vi "InjB-RT.vi"() -> ()   [LabVIEW 2016]
uses:
  <vilib>/rvi/interface/nirviOpenFPGA/nirviOpenFPGA.xnode
  InjB-FPGA.vi
  <vilib>/rvi/interface/nirviReadWriteControl/nirviReadWriteControl.xnode
  HV Readbacks.ctl
  RT ctls.lvlib
  <vilib>/Utility/error.llb/Error Cluster From Error Code.vi
  <vilib>/rvi/interface/Simulation/niFpgaSimulationCallBeginRW.vi
  <vilib>/rvi/errors/niLvFpgaAdjustHostInterfaceError.vi
  Aperture RT Readbacks.ctl
  <vilib>/platform/TimedLoop/XDataNode/XDataNode.xnode
  <vilib>/Platform/TimedLoop/XDataNode/nitl_modes.ctl
  <vilib>/Platform/TimedLoop/XDataNode/XDNodeRunTimeDep.lvlib
  <vilib>/Platform/TimedLoop/XDataNode/wakeup.ctl
  <vilib>/Platform/TimedLoop/XDataNode/timing_clust.ctl
  Glassman Control.ctl
  NiFpgaLv.dll
  Pressure Gauge.ctl
  HV Controls.ctl
  Aperture RT Controls.ctl
panel:
  out "Cryo ON-Time RAW":string
  out "Cryo 1st Stage Temperature RAW":string
  out "Cryo 1st Stage Temperature":string
  out "Cryo ON-Time":string
  out "Cryo Status":string
  out "Cryo Status RAW":string
  out "Beamline":T1
  out "Ion Source":T1
  out "Ion Source IG2":dbl
  out "Ion Source CG2":dbl
  out "Ion Source CG1":dbl
  out "Ion Source IG1":dbl
  out "Beamline IG1":dbl
  out "Beamline CG1":dbl
  out "Beamline IG2":dbl
  out "Beamline CG2":dbl
  in  "Injector Aperture Controls":T2
  in  "Injector HV Controls":T3
  out "Injector Aperture Readbacks":T4
  out "Injector HV Readbacks":T5
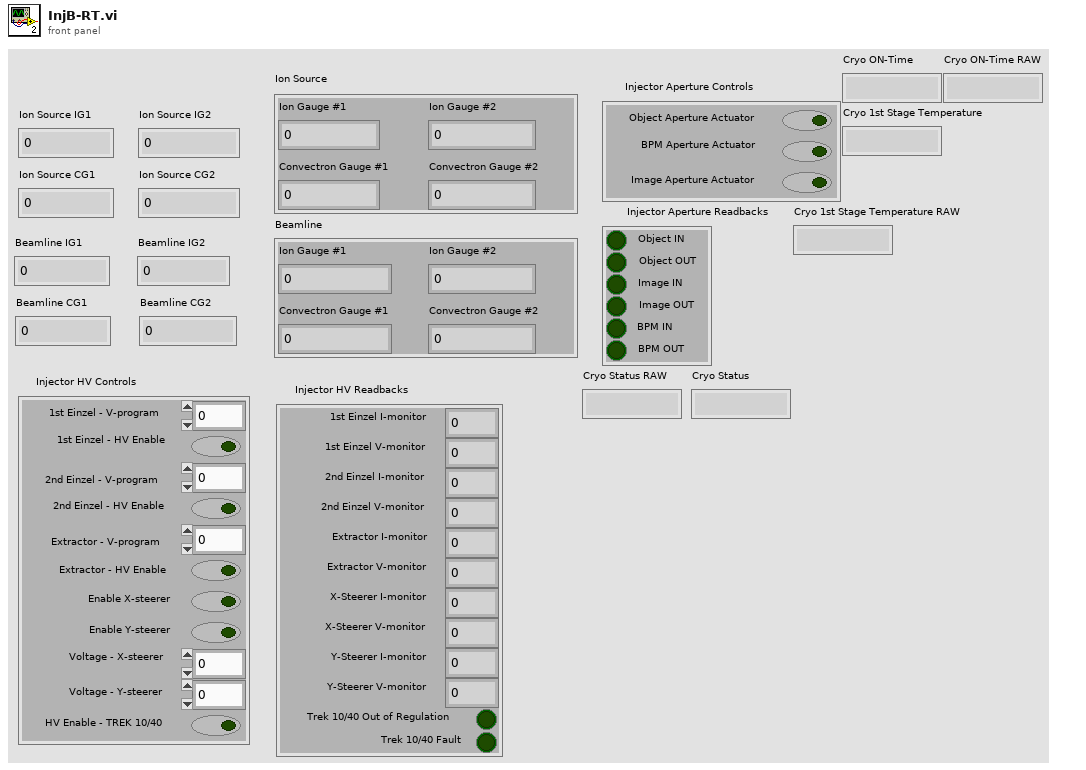
[diagram p1: front panel]
types:
  T1 = typedef "Pressure Gauge.ctl" = cluster{"Ion Gauge #1":dbl, "Convectron Gauge #1":dbl, "Convectron Gauge #2":dbl, "Ion Gauge #2":dbl}
  T2 = typedef "RT ctls.lvlib/Aperture RT Controls.ctl" = cluster{"Object Aperture Actuator":bool, "BPM Aperture Actuator":bool, "Image Aperture Actuator":bool}
  T3 = typedef "RT ctls.lvlib/HV Controls.ctl" = cluster{"Enable X-steerer":bool, "Enable Y-steerer":bool, "Voltage - X-steerer":fxp<+/-,20,5>, "Voltage - Y-steerer":fxp<+/-,20,5>, "HV Enable - TREK 10/40":bool, "1st Einzel - V-program":fxp<+/-,20,5>, "1st Einzel - HV Enable":bool, "2nd Einzel - V-program":fxp<+/-,20,5>, "2nd Einzel - HV Enable":bool, "Extractor - V-program":fxp<+/-,20,5>, "Extractor - HV Enable":bool}
  T4 = typedef "RT ctls.lvlib/Aperture RT Readbacks.ctl" = cluster{"Object IN":bool, "Object OUT":bool, "Image IN":bool, "Image OUT":bool, "BPM IN":bool, "BPM OUT":bool}
  T5 = typedef "RT ctls.lvlib/HV Readbacks.ctl" = cluster{"1st Einzel I-monitor":fxp<+/-,26,5>, "1st Einzel V-monitor":fxp<+/-,26,5>, "2nd Einzel I-monitor":fxp<+/-,26,5>, "2nd Einzel V-monitor":fxp<+/-,26,5>, "Extractor I-monitor":fxp<+/-,26,5>, "Extractor V-monitor":fxp<+/-,26,5>, "X-Steerer I-monitor":fxp<+/-,26,5>, "X-Steerer V-monitor":fxp<+/-,26,5>, "Y-Steerer I-monitor":fxp<+/-,26,5>, "Y-Steerer V-monitor":fxp<+/-,26,5>, "Trek 10/40 Out of Regulation":bool, "Trek 10/40 Fault":bool}
  T6 = typedef "XDNodeRunTimeDep.lvlib/timing_clust.ctl" = cluster{"Expected End [f-1]":u64, "Actual End [f-1]":u64, "Finished Late? [f-1]":bool, "Expected End [i-1]":u64, "Actual End [i-1]":u64, "Finished Late? [i-1]":bool, "Expected Start [i]":u64, "Actual Start [i]":u64, "Expected Start [f]":u64, "Actual Start [f]":u64, "Source Name":string, "Structure Name":string, "Period":i64, "Deadline":i64, "Offset":i64, "Start":i64, "Priority":i32, "Timeout":i32, "Mode":T7, "Wakeup Reason":T8, "Error":errorcluster, "Source Type":string, "Secondary Source Type":string, "Global End Time":u64, "Global Start Time":u64, "Frame Duration":u64, "Iteration Duration":u64, "Assigned CPU":i32, "I/O Scan Engine Mode":u32}
  T7 = typedef "XDNodeRunTimeDep.lvlib/nitl_modes.ctl" = enum32{"No Change", "Process missed periods, maintain original phase", "Discard missed periods, maintain original phase", "Process missed periods, ignore original phase", "Discard missed periods, ignore original phase"}
  T8 = typedef "XDNodeRunTimeDep.lvlib/wakeup.ctl" = enum32{"Normal", "Aborted", "Asynchronous wakeup", "Timing source error", "Timed loop error", "Timeout"}
  T9 = cluster{"I-monitor":fxp<+/-,26,5>, "V-monitor":fxp<+/-,26,5>}
  T10 = typedef "Glassman Control.ctl" = cluster{"V-program":fxp<+/-,20,5>, "HV Enable":bool}
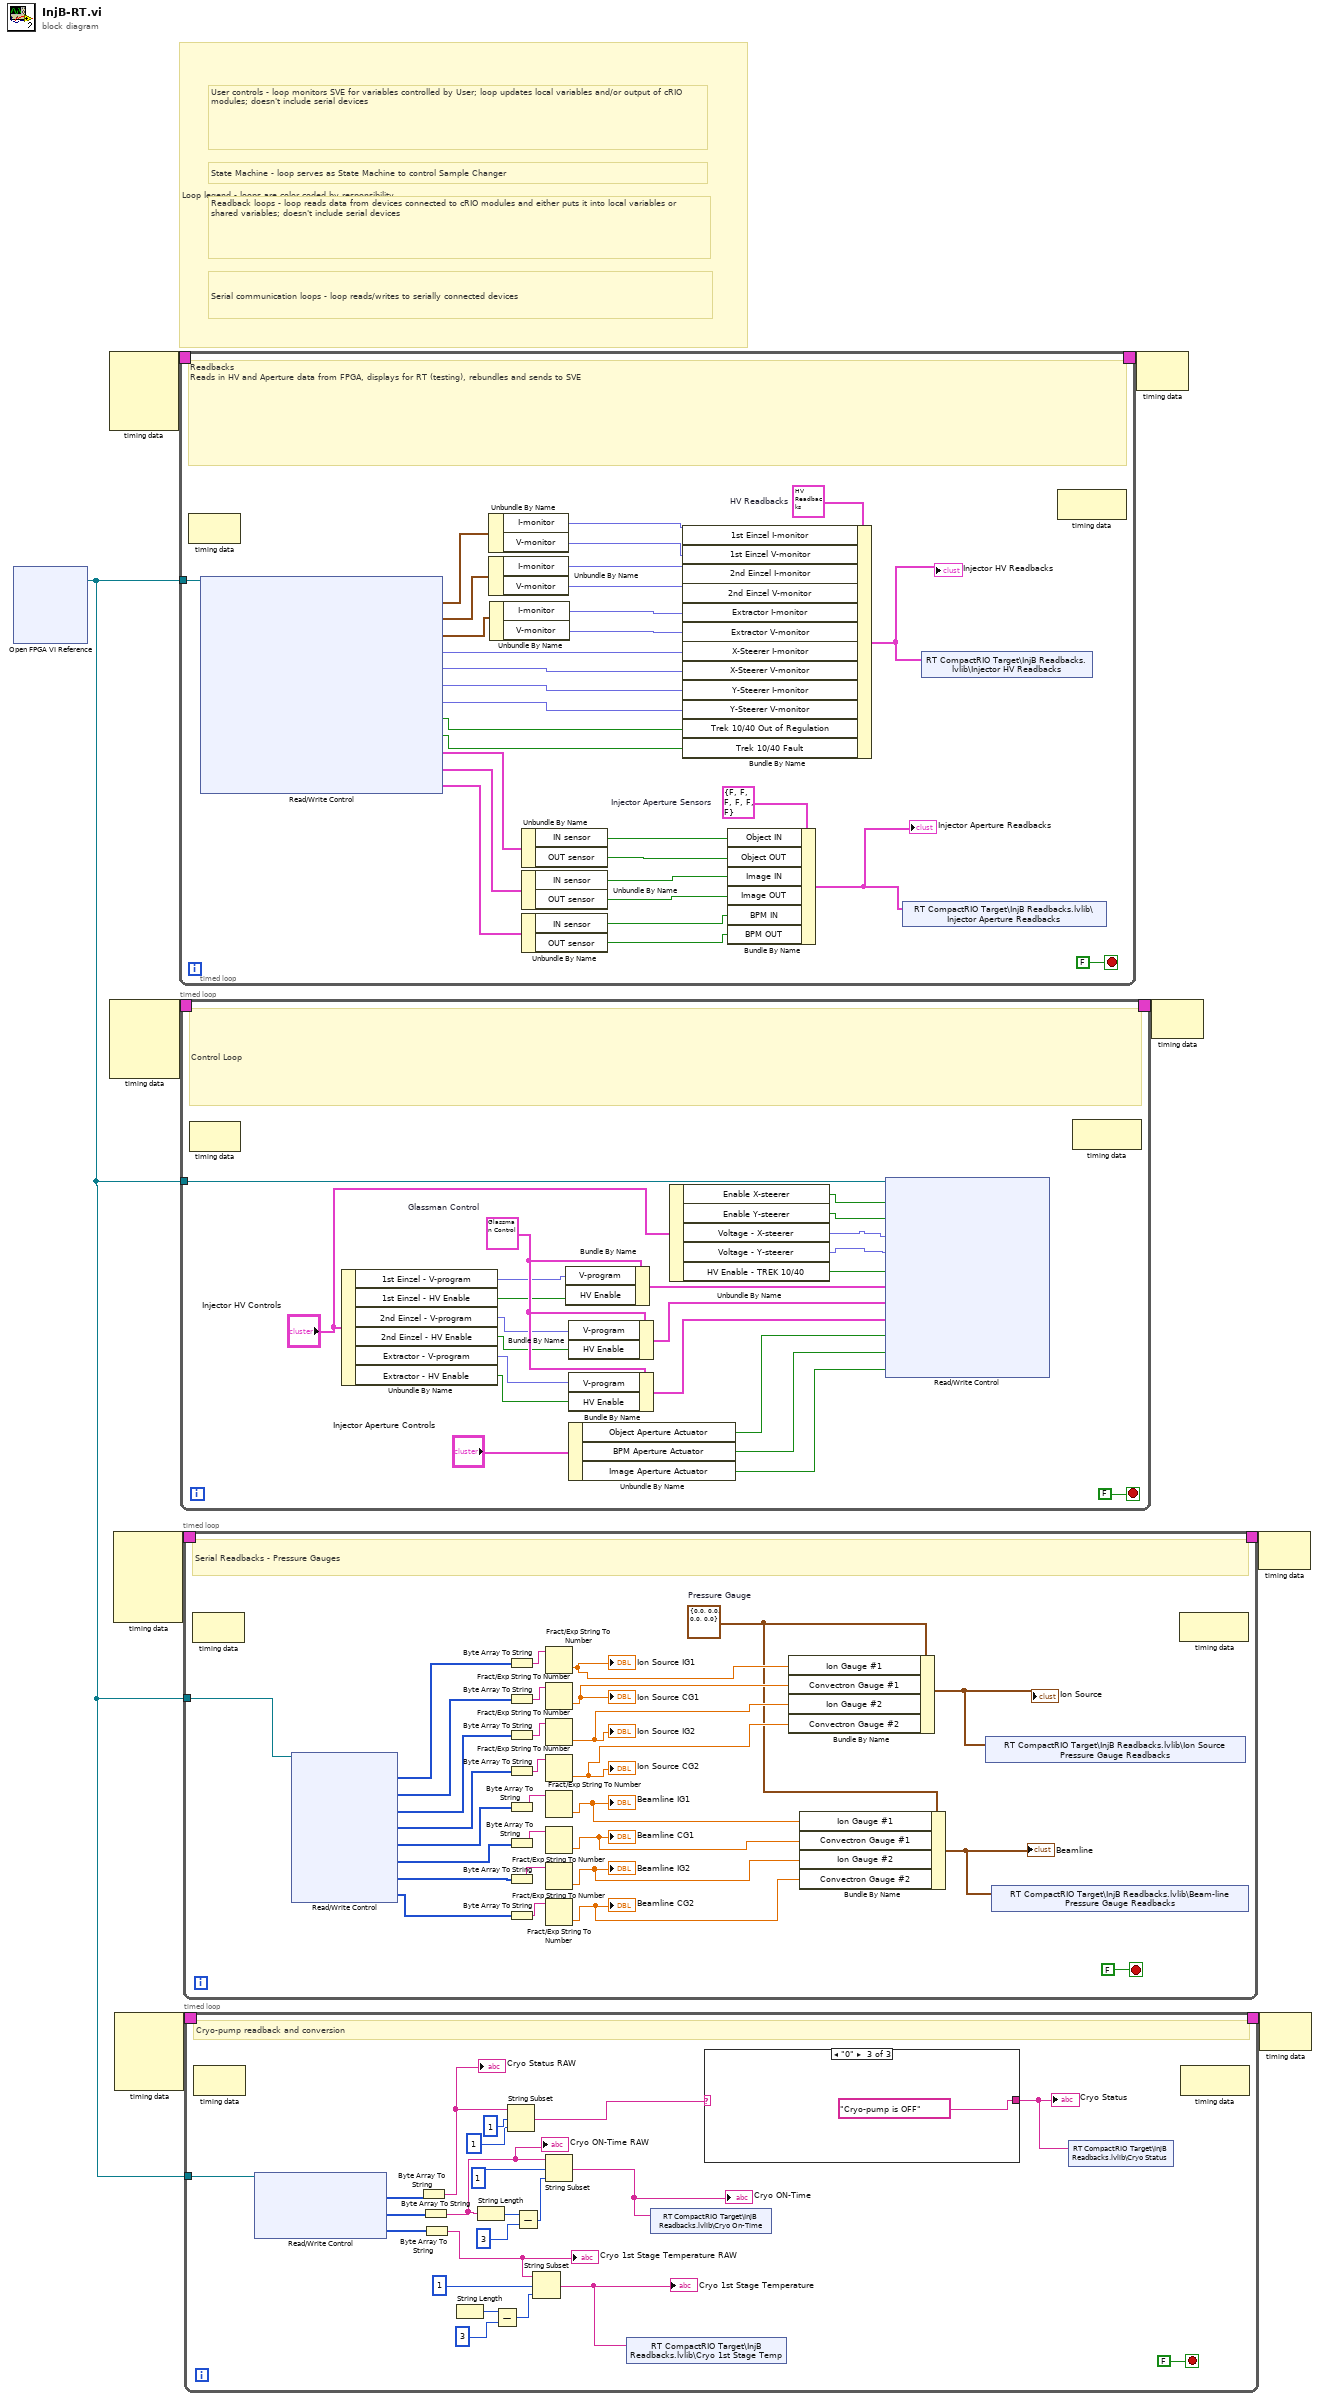
[diagram p0: block diagram]
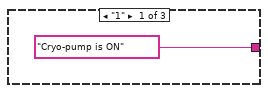
[diagram p2: hidden frame]
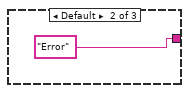
[diagram p3: hidden frame]
diagram:
  # "Serial communication loops - loop reads/writes to serially connected devices"
  # "Readback loops - loop reads data from devices connected to cRIO modules and either puts it into local variables or shared variables; doesn't include serial devices"
  # "State Machine - loop serves as State Machine to control Sample Changer"
  # "User controls - loop monitors SVE for variables controlled by User; loop updates local variables and/or output of cRIO modules; doesn't include serial devices"
  # "Loop legend - loops are color coded by responsibility"
  n1 = xnode "Open FPGA VI Reference"() -> ("FPGA VI Reference Out"=w1:refnum<k20>)  [unwired: 2 in, 1 out]
  n2 = node-c288() -> (w9:T6)  [unwired: 4 in]
  n3 = node-c288() -> (w7:T6)  [unwired: 4 in]
  n4 = node-c288() -> (w5:T6)  [unwired: 5 in]
  n5 = node-c288() -> (w3:T6)  [unwired: 4 in]
  n6 = timed-loop {
    tunnel: w1 -> [w39]
    timing: w9 -> [_]
    timing-out: [_] -> w8
    stop <- FALSE stop-if-true
    w18 = T4 {"Object IN"=FALSE, "Object OUT"=FALSE, "Image IN"=FALSE, "Image OUT"=FALSE, "BPM IN"=FALSE, "BPM OUT"=FALSE}  # Injector Aperture Sensors
    w38 = T5 {"1st Einzel I-monitor"=0.0, "1st Einzel V-monitor"=0.0, "2nd Einzel I-monitor"=0.0, "2nd Einzel V-monitor"=0.0, "Extractor I-monitor"=0.0, "Extractor V-monitor"=0.0, "X-Steerer I-monitor"=0.0, "X-Steerer V-monitor"=0.0, "Y-Steerer I-monitor"=0.0, "Y-Steerer V-monitor"=0.0, "Trek 10/40 Out of Regulation"=FALSE, "Trek 10/40 Fault"=FALSE}  # HV Readbacks
    # "Readbacks\nReads in HV and Aperture data from FPGA, displays for RT (testing), rebundles and sends to SVE"
    n7 = node-c288() -> ()  [unwired: 1 in, 1 out]
    n8 = xnode "Read/Write Control"("FPGA VI Reference In"=w39) -> ("1st Einzel"=w25:T9, "2nd Einzel"=w26:T9, "Extractor"=w27:T9, "I-monitor - X-steerer"=w31:fxp<+/-,26,5>, "V-monitor - X-steerer"=w30:fxp<+/-,26,5>, "I-monitor - Y-steerer"=w29:fxp<+/-,26,5>, "V-monitor - Y-steerer"=w28:fxp<+/-,26,5>, "Out-of-Regulation Status - TREK 10/40"=w24:bool, "Fault Status - TREK 10/40"=w23:bool, "Object Aperture Sensors"=w21:cluster{"IN sensor":bool, "OUT sensor":bool}, "Image Aperture Sensors"=w20:cluster{"IN sensor":bool, "OUT sensor":bool}, "BPM Aperture Sensors"=w19:cluster{"IN sensor":bool, "OUT sensor":bool})  [unwired: 1 in, 2 out]
    n9 = Unbundle By Name(w25) -> ("I-monitor"=w32:fxp<+/-,26,5>, "V-monitor"=w33:fxp<+/-,26,5>)
    n10 = Unbundle By Name(w26) -> ("I-monitor"=w34:fxp<+/-,26,5>, "V-monitor"=w35:fxp<+/-,26,5>)
    n11 = Unbundle By Name(w27) -> ("I-monitor"=w36:fxp<+/-,26,5>, "V-monitor"=w37:fxp<+/-,26,5>)
    n12 = Unbundle By Name(w21) -> ("IN sensor"=w17:bool, "OUT sensor"=w16:bool)
    n13 = Unbundle By Name(w20) -> ("IN sensor"=w15:bool, "OUT sensor"=w14:bool)
    n14 = Unbundle By Name(w19) -> ("IN sensor"=w13:bool, "OUT sensor"=w12:bool)
    n15 = Bundle By Name(cluster=w38, "1st Einzel I-monitor"=w32, "1st Einzel V-monitor"=w33, "2nd Einzel I-monitor"=w34, "2nd Einzel V-monitor"=w35, "Extractor I-monitor"=w36, "Extractor V-monitor"=w37, "X-Steerer I-monitor"=w31, "X-Steerer V-monitor"=w30, "Y-Steerer I-monitor"=w29, "Y-Steerer V-monitor"=w28, "Trek 10/40 Out of Regulation"=w24, "Trek 10/40 Fault"=w23) -> (w10:T5)
    "Injector HV Readbacks" <- w10
    n16 = Bundle By Name(cluster=w18, "Object IN"=w17, "Object OUT"=w16, "Image IN"=w15, "Image OUT"=w14, "BPM IN"=w13, "BPM OUT"=w12) -> (w11:T4)
    "Injector Aperture Readbacks" <- w11
    n17 = shared-variable "RT CompactRIO Target\\InjB Readbacks.lvlib\\Injector Aperture Readbacks"(w11) -> ()  [unwired: 1 in, 1 out]
    n18 = shared-variable "RT CompactRIO Target\\InjB Readbacks.lvlib\\Injector HV Readbacks"(w10) -> ()  [unwired: 1 in, 1 out]
    n19 = node-c288() -> ()  [unwired: 1 in, 1 out]
  }
  n20 = timed-loop {
    timing: w7 -> [_]
    timing-out: [_] -> w6
    tunnel: w1 -> [w62]
    stop <- FALSE stop-if-true
    w58 = T10 {"V-program"=0.0, "HV Enable"=FALSE}  # Glassman Control
    # "Control Loop"
    n21 = node-c288() -> ()  [unwired: 1 in, 1 out]
    n22 = Unbundle By Name("Injector HV Controls") -> ("1st Einzel - V-program"=w51:fxp<+/-,20,5>, "1st Einzel - HV Enable"=w50:bool, "2nd Einzel - V-program"=w49:fxp<+/-,20,5>, "2nd Einzel - HV Enable"=w48:bool, "Extractor - V-program"=w47:fxp<+/-,20,5>, "Extractor - HV Enable"=w46:bool)
    n23 = Bundle By Name(cluster=w58, "V-program"=w51, "HV Enable"=w50) -> (w61:T10)
    n24 = Unbundle By Name("Injector Aperture Controls") -> ("Object Aperture Actuator"=w44:bool, "BPM Aperture Actuator"=w43:bool, "Image Aperture Actuator"=w42:bool)
    n25 = Bundle By Name(cluster=w58, "V-program"=w49, "HV Enable"=w48) -> (w60:T10)
    n26 = Bundle By Name(cluster=w58, "V-program"=w47, "HV Enable"=w46) -> (w59:T10)
    n27 = Unbundle By Name("Injector HV Controls") -> ("Enable X-steerer"=w53:bool, "Enable Y-steerer"=w57:bool, "Voltage - X-steerer"=w56:fxp<+/-,20,5>, "Voltage - Y-steerer"=w55:fxp<+/-,20,5>, "HV Enable - TREK 10/40"=w54:bool)
    n28 = xnode "Read/Write Control"("FPGA VI Reference In"=w62, "Enable X-steerer"=w53, "Enable Y-steerer"=w57, "Voltage - X-steerer"=w56, "Voltage - Y-steerer"=w55, "HV Enable - TREK 10/40"=w54, "1st Einzel Control"=w61, "2nd Einzel Control"=w60, "Extractor Control"=w59, "Object Aperture Actuator"=w44, "BPM Aperture Actuator"=w43, "Image Aperture Actuator"=w42) -> ()  [unwired: 1 in, 2 out]
    n29 = node-c288() -> ()  [unwired: 1 in, 1 out]
  }
  n30 = timed-loop {
    timing: w5 -> [_]
    timing-out: [_] -> w4
    tunnel: w1 -> [w92]
    stop <- FALSE stop-if-true
    w71 = T1 {"Ion Gauge #1"=0.0, "Convectron Gauge #1"=0.0, "Convectron Gauge #2"=0.0, "Ion Gauge #2"=0.0}  # Pressure Gauge
    # "Serial Readbacks - Pressure Gauges"
    n31 = node-c288() -> ()  [unwired: 1 in, 1 out]
    n32 = xnode "Read/Write Control"("FPGA VI Reference In"=w92) -> ("Ion Source IG1"=w94:u8[], "Ion Source CG1"=w83:u8[], "Ion Source IG2"=w82:u8[], "Ion Source CG2"=w81:u8[], "Beamline IG1"=w80:u8[], "Beamline CG1"=w79:u8[], "Beamline IG2"=w78:u8[], "Beamline CG2"=w77:u8[])  [unwired: 1 in, 2 out]
    n33 = Byte Array To String(unsigned byte array=w94) -> (string=w91:string)
    n34 = Byte Array To String(unsigned byte array=w83) -> (string=w90:string)
    n35 = Byte Array To String(unsigned byte array=w82) -> (string=w89:string)
    n36 = Byte Array To String(unsigned byte array=w81) -> (string=w88:string)
    n37 = Byte Array To String(unsigned byte array=w80) -> (string=w87:string)
    n38 = Byte Array To String(unsigned byte array=w79) -> (string=w86:string)
    n39 = Byte Array To String(unsigned byte array=w78) -> (string=w85:string)
    n40 = Byte Array To String(unsigned byte array=w77) -> (string=w84:string)
    n41 = Fract/Exp String To Number(string=w91) -> (number=w75:dbl)  [unwired: 3 in, 1 out]
    "Ion Source IG1" <- w75
    n42 = Fract/Exp String To Number(string=w90) -> (number=w74:dbl)  [unwired: 3 in, 1 out]
    "Ion Source CG1" <- w74
    n43 = Fract/Exp String To Number(string=w89) -> (number=w73:dbl)  [unwired: 3 in, 1 out]
    "Ion Source IG2" <- w73
    n44 = Fract/Exp String To Number(string=w88) -> (number=w72:dbl)  [unwired: 3 in, 1 out]
    "Ion Source CG2" <- w72
    n45 = Fract/Exp String To Number(string=w87) -> (number=w70:dbl)  [unwired: 3 in, 1 out]
    "Beamline IG1" <- w70
    n46 = Fract/Exp String To Number(string=w86) -> (number=w69:dbl)  [unwired: 3 in, 1 out]
    "Beamline CG1" <- w69
    n47 = Fract/Exp String To Number(string=w85) -> (number=w68:dbl)  [unwired: 3 in, 1 out]
    "Beamline IG2" <- w68
    n48 = Fract/Exp String To Number(string=w84) -> (number=w67:dbl)  [unwired: 3 in, 1 out]
    "Beamline CG2" <- w67
    n49 = Bundle By Name(cluster=w71, "Ion Gauge #1"=w75, "Convectron Gauge #1"=w74, "Ion Gauge #2"=w73, "Convectron Gauge #2"=w72) -> (w76:T1)
    "Ion Source" <- w76
    n50 = Bundle By Name(cluster=w71, "Ion Gauge #1"=w70, "Convectron Gauge #1"=w69, "Ion Gauge #2"=w68, "Convectron Gauge #2"=w67) -> (w66:T1)
    "Beamline" <- w66
    n51 = shared-variable "RT CompactRIO Target\\InjB Readbacks.lvlib\\Ion Source Pressure Gauge Readbacks"(w76) -> ()  [unwired: 1 in, 1 out]
    n52 = shared-variable "RT CompactRIO Target\\InjB Readbacks.lvlib\\Beam-line Pressure Gauge Readbacks"(w66) -> ()  [unwired: 1 in, 1 out]
    n53 = node-c288() -> ()  [unwired: 1 in, 1 out]
  }
  n54 = timed-loop "Timed Loop" {
    timing: w3 -> [_]
    timing-out: [_] -> w2
    tunnel: w1 -> [w117]
    stop <- FALSE stop-if-true
    # "Cryo-pump readback and conversion"
    n55 = node-c288() -> ()  [unwired: 1 in, 1 out]
    n56 = xnode "Read/Write Control"("FPGA VI Reference In"=w117) -> ("Cryo status"=w116:u8[], "Cryo On-time"=w115:u8[], "Cryo 1st stage temp"=w114:u8[])  [unwired: 1 in, 2 out]
    n57 = Byte Array To String(unsigned byte array=w116) -> (string=w113:string)
    "Cryo Status RAW" <- w113
    n58 = Byte Array To String(unsigned byte array=w115) -> (string=w108:string)
    "Cryo ON-Time RAW" <- w108
    n59 = Byte Array To String(unsigned byte array=w114) -> (string=w99:string)
    "Cryo 1st Stage Temperature RAW" <- w99
    n60 = String Length() -> (length=w102:i32)  [unwired: 1 in]
    n61 = String Length(string=w108) -> (length=w107:i32)
    n62 = Subtract(x=w102, y=3) -> (x-y=w100:i32)
    n63 = String Subset(string=w113, offset (0)=1, length (rest)=1 ("length (rest)")) -> (substring=w109:string)
    n64 = Subtract(x=w107, y=3) -> (x-y=w105:i32)
    n65 = String Subset(string=w99, offset (0)=1, length (rest)=w100) -> (substring=w97:string)
    "Cryo 1st Stage Temperature" <- w97
    n66 = String Subset(string=w108, offset (0)=1, length (rest)=w105) -> (substring=w103:string)
    "Cryo ON-Time" <- w103
    n67 = shared-variable "RT CompactRIO Target\\InjB Readbacks.lvlib\\Cryo 1st Stage Temp"(w97) -> ()  [unwired: 1 in, 1 out]
    n68 = shared-variable "RT CompactRIO Target\\InjB Readbacks.lvlib\\Cryo On-Time"(w103) -> ()  [unwired: 1 in, 1 out]
    n69 = case shown="\"0\"" w109 {
      tunnel: ["Cryo-pump is ON" "Error" "Cryo-pump is OFF"] -> w104
      frame "1" {
      }
      frame Default {
      }
      frame "0" {
      }
    }
    "Cryo Status" <- w104
    n70 = shared-variable "RT CompactRIO Target\\InjB Readbacks.lvlib\\Cryo Status"(w104) -> ()  [unwired: 1 in, 1 out]
    n71 = node-c288() -> ()  [unwired: 1 in, 1 out]
  }
  n72 = node-c288(w8) -> ()  [unwired: 1 out]
  n73 = node-c288(w6) -> ()  [unwired: 1 out]
  n74 = node-c288(w4) -> ()  [unwired: 1 out]
  n75 = node-c288(w2) -> ()  [unwired: 1 out]
